vi "PeelingMXIDaily.vi"() -> ()   [LabVIEW 2012]
uses:
  <vilib>/addons/database/Connection.llb/DB Tools Open Connec (Path).vi
  <vilib>/addons/database/Connection.llb/Conn Execute.vi
  <vilib>/addons/database/Recordset.llb/Rec Fetch Recordset Data (R).vi
  <vilib>/addons/database/Recordset.llb/Rec Destroy - Connection.vi
  <vilib>/Utility/file.llb/Write To Spreadsheet File (string).vi
  <vilib>/addons/database/_DB Variant To Data/Database Variant To Data.xnode
  <vilib>/addons/database/NI_Database_API.lvlib
panel:
  out "error out":errorcluster
  out "Array 2":string[][](array[string])
  out "spreadsheet string":string
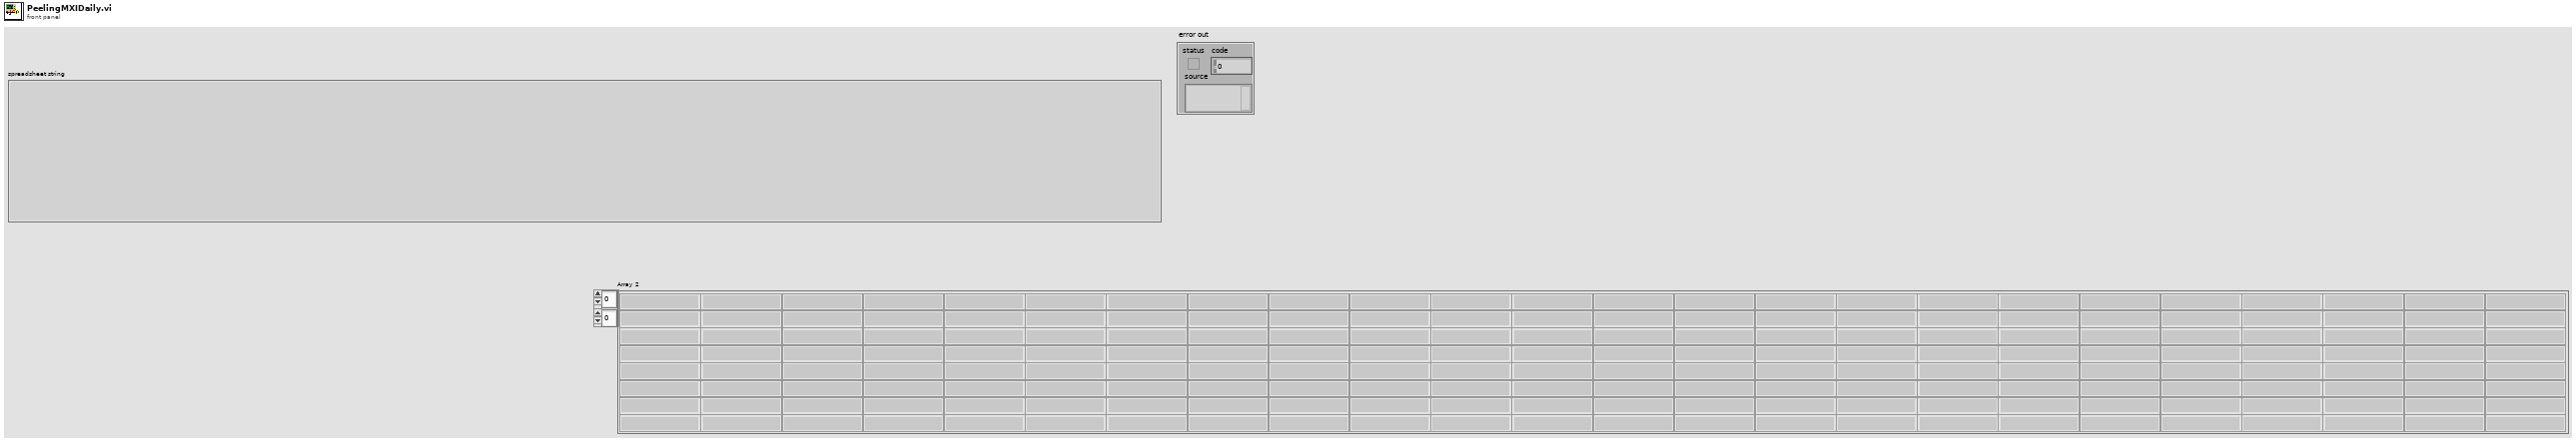
[diagram p1: front panel]
types:
  T1 = typedef "NI_Database_API.lvlib/Conn ObjectReference.ctl" = refnum<k1>
  T2 = typedef "NI_Database_API.lvlib/Rec ObjectReference.ctl" = refnum<k1>
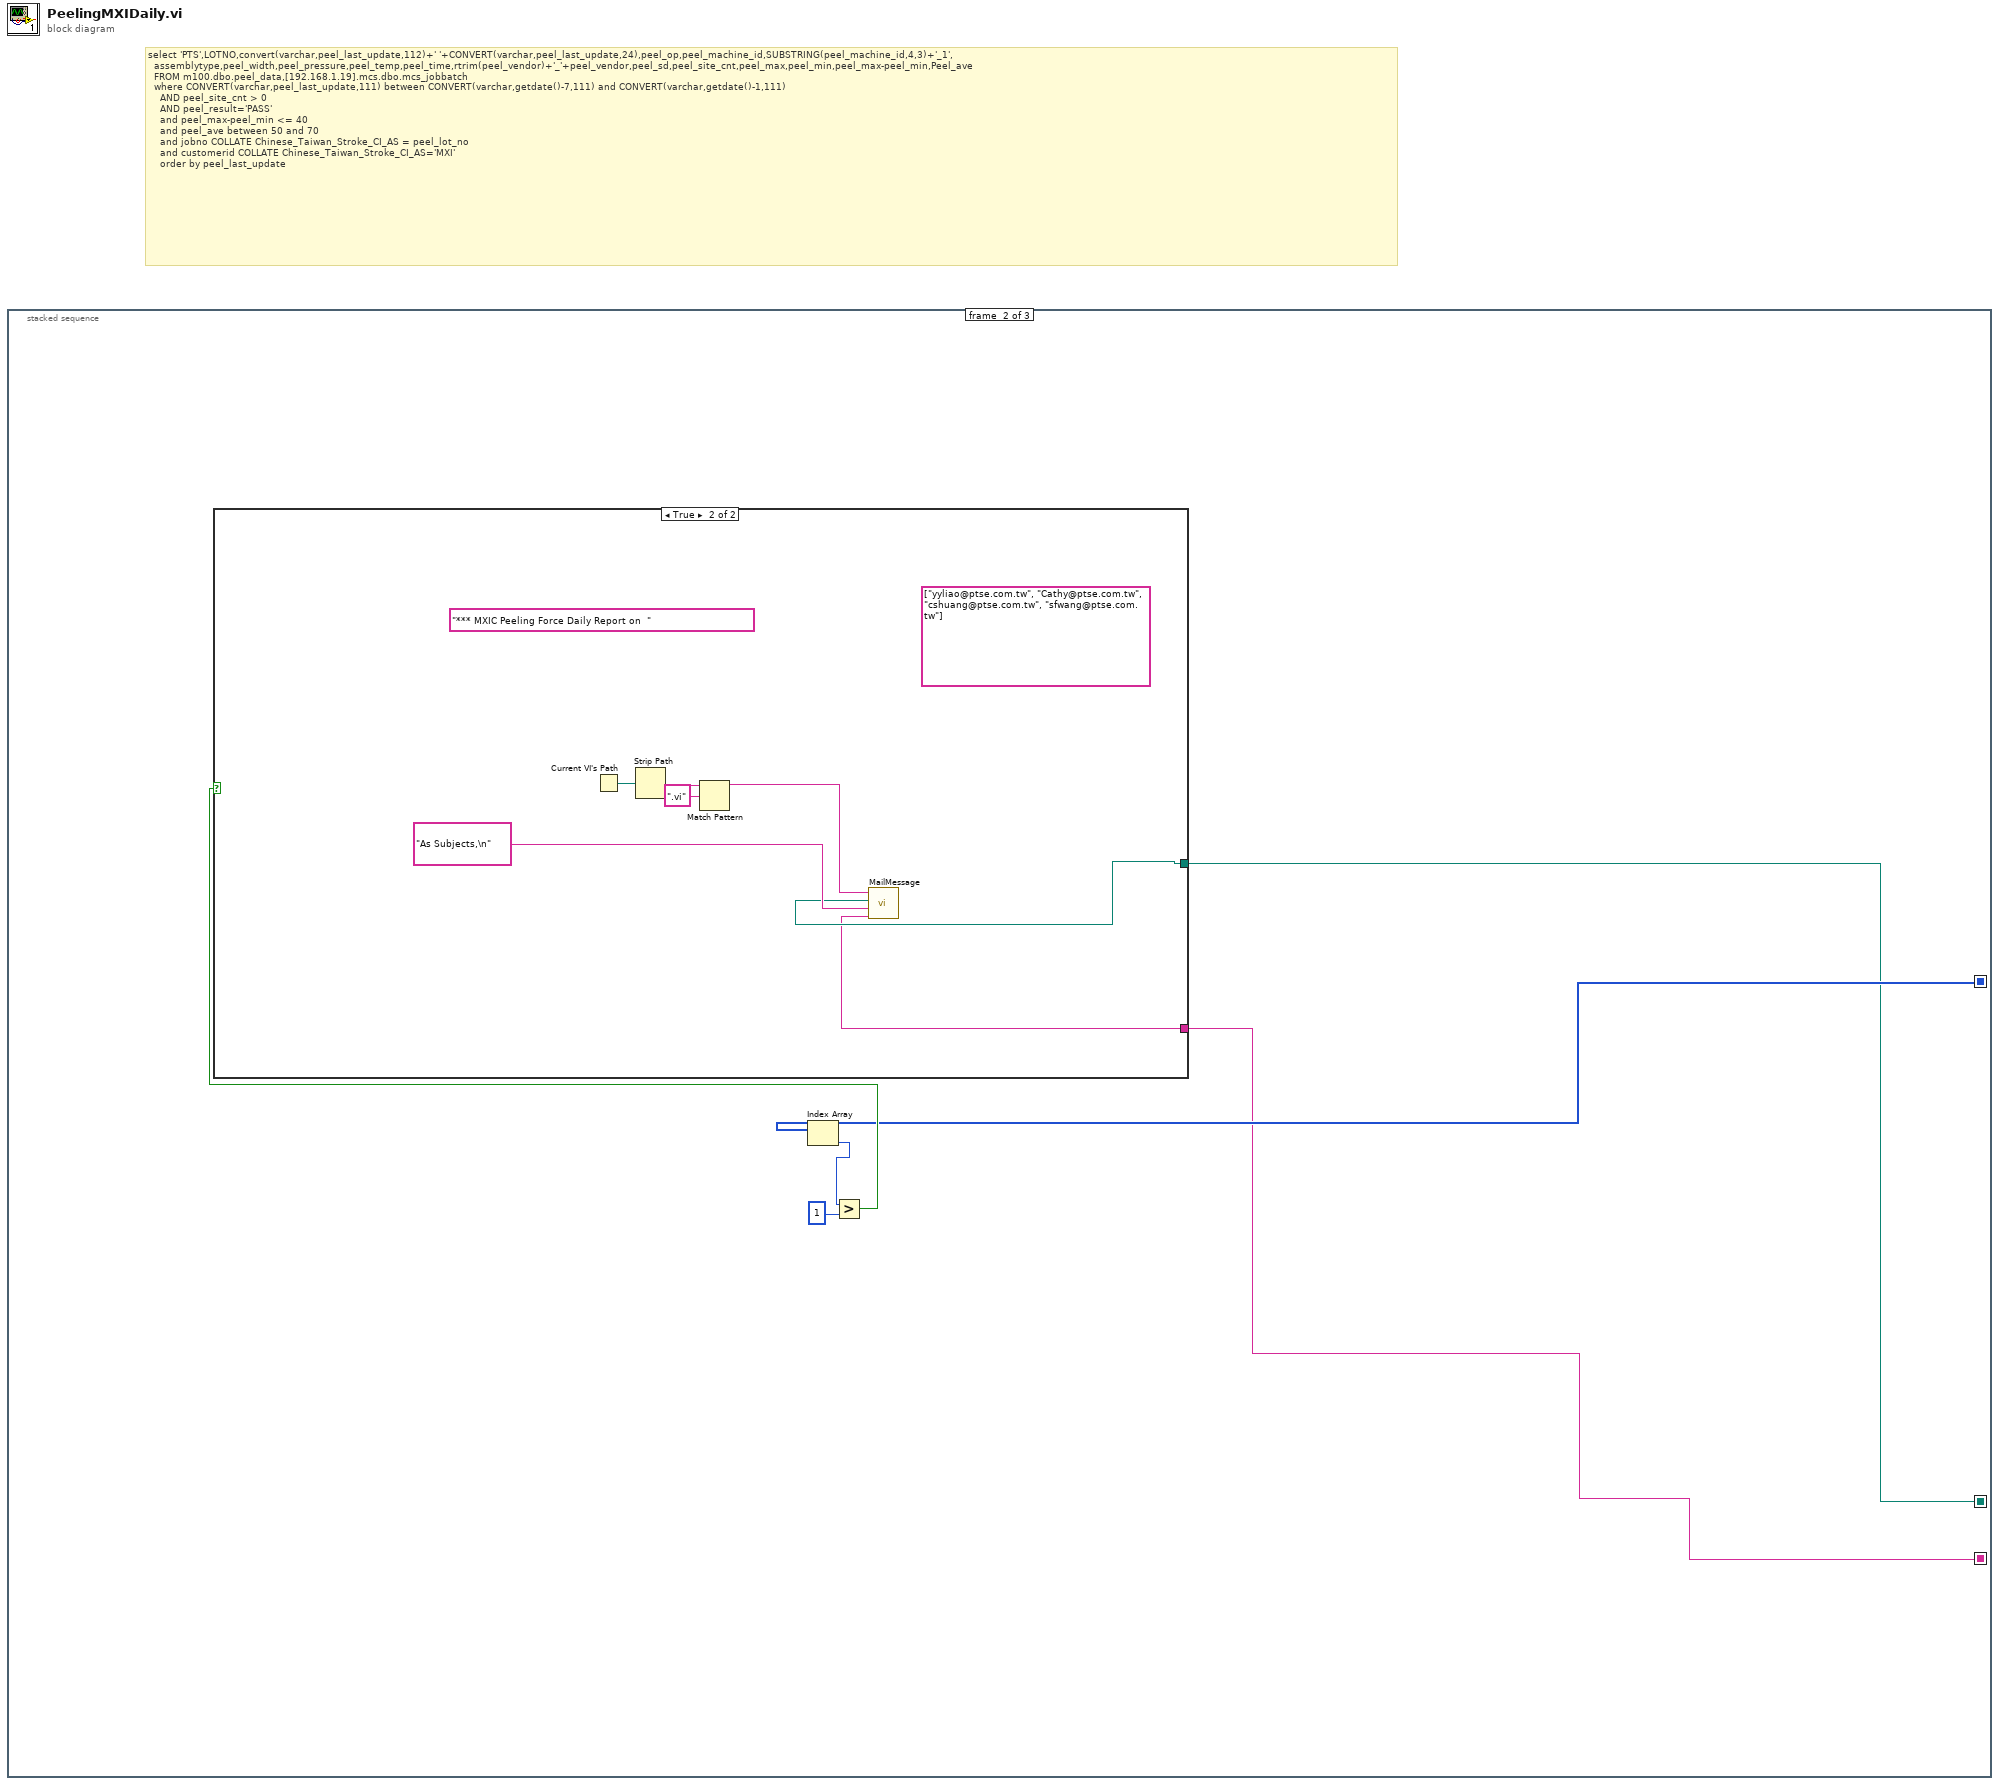
[diagram p0: block diagram]
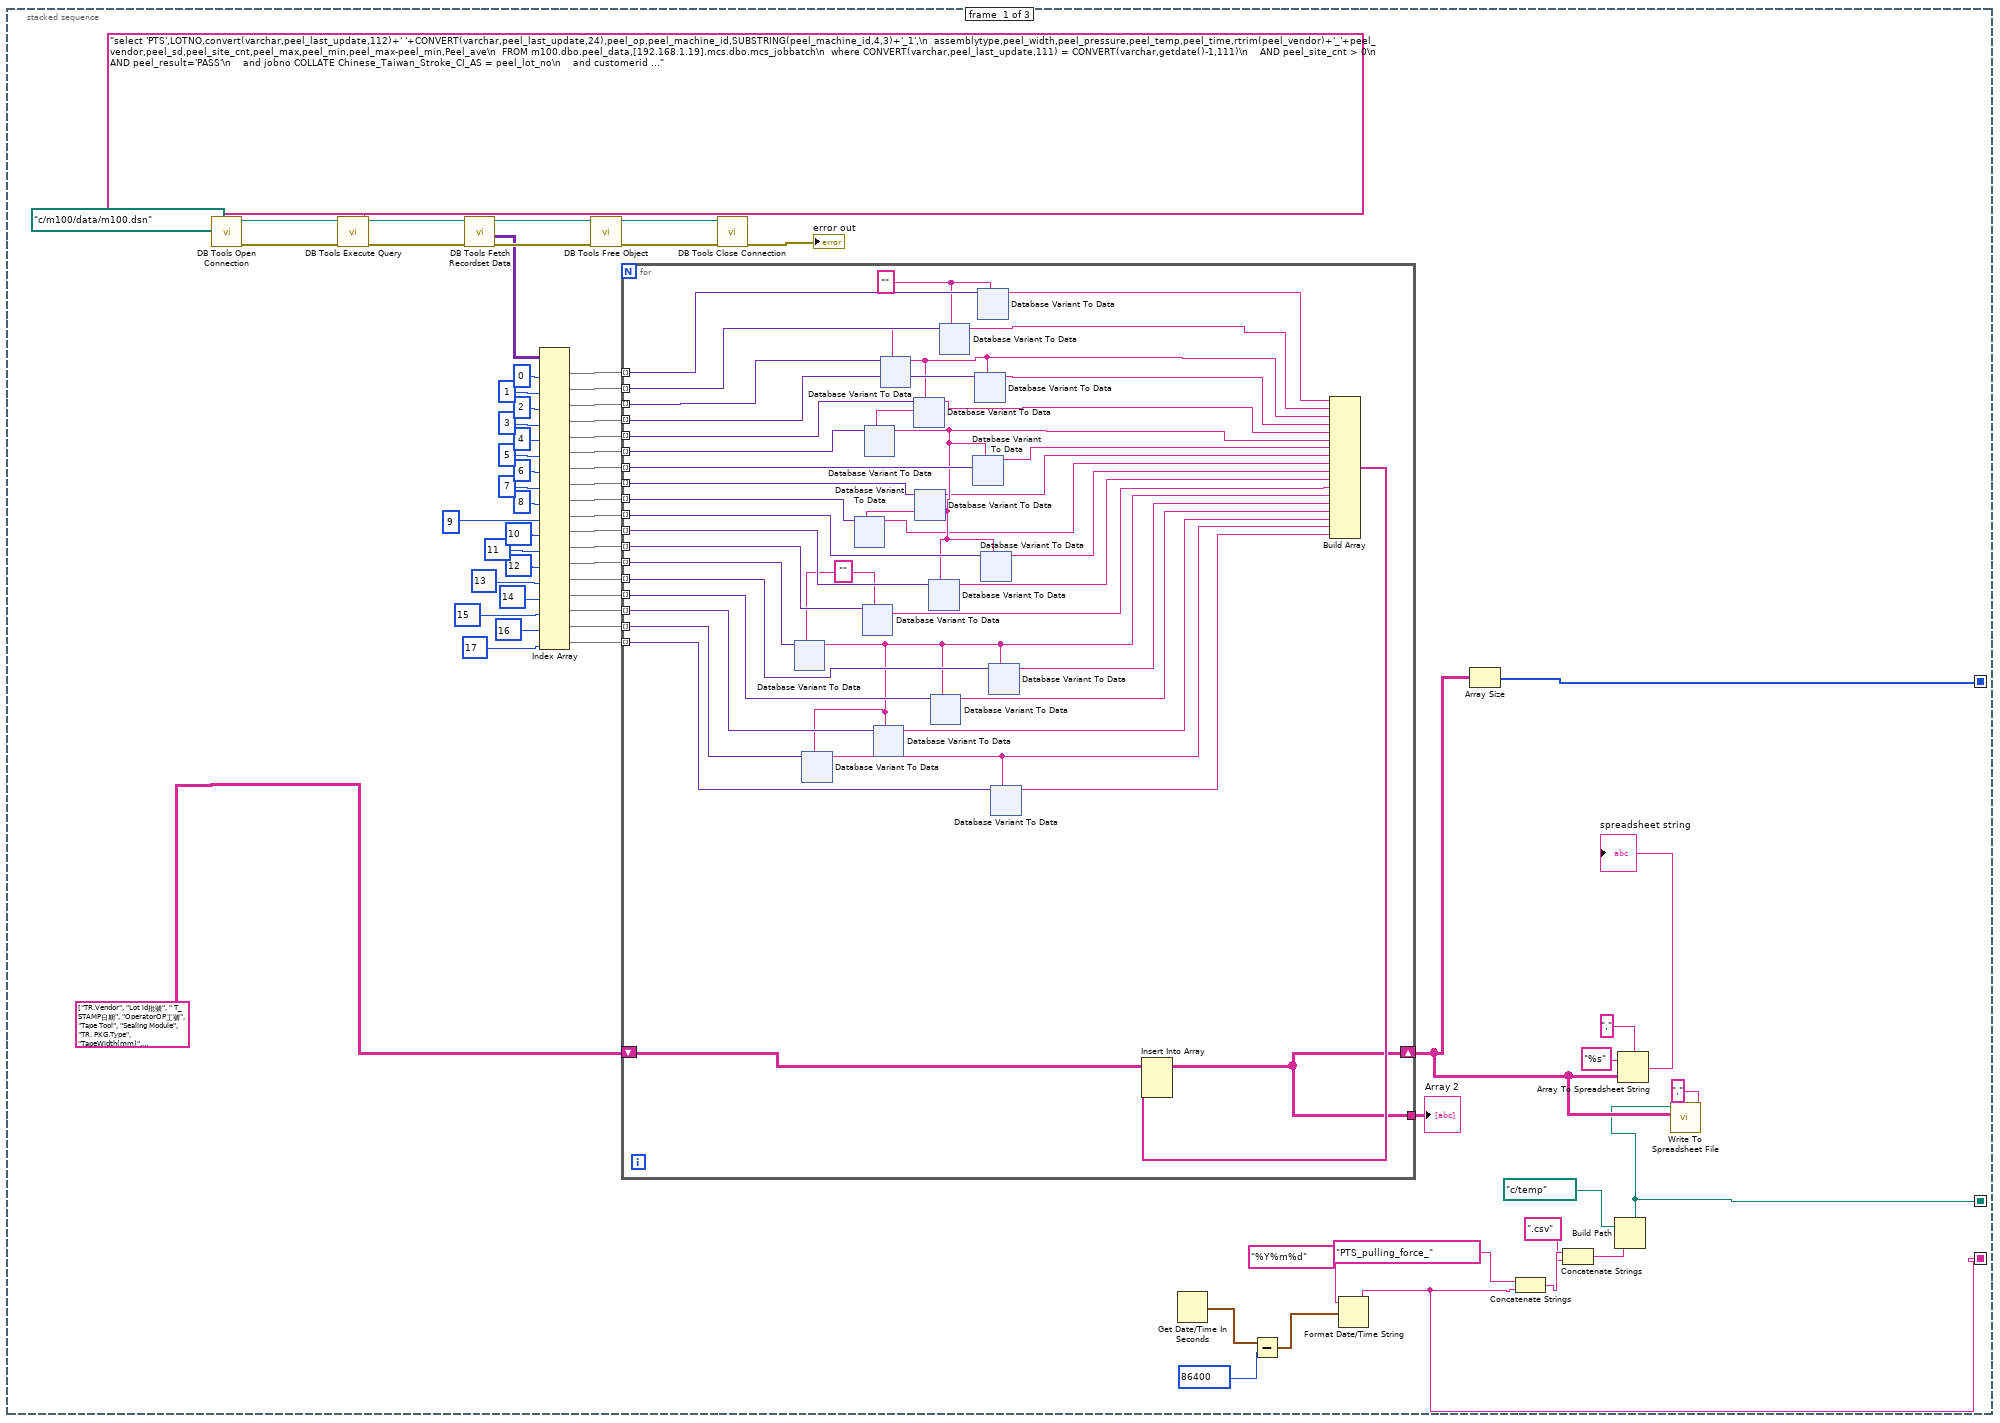
[diagram p2: hidden frame]
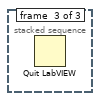
[diagram p4: hidden frame]
diagram:
  # "select 'PTS',LOTNO,convert(varchar,peel_last_update,112)+' '+CONVERT(varchar,peel_last_update,24),peel_op,peel_machine_id,SUBSTRING(peel_machine_id,4,3)+'_1',\n  assemblytype,peel_width,peel_pressure,peel_temp,peel_time,rtrim(peel_vendor)+'_'+peel_vendor,peel_sd,peel_site_cnt,peel_max,peel_min,peel_max-peel_min,Peel_ave\n  FROM m100.dbo.peel_data,[192.168.1.19].mcs.dbo.mcs_jobbatch\n  where CONVERT(varchar,peel_last_update,111) between CONVERT(varchar,getdate()-7,111) and CONVERT(varchar,getdate()-1,111)\n    AND peel_site_cnt > 0\n    AND peel_result='PASS'\n    and peel_max-peel_min <= 40\n    and peel_ave between 50 and 70\n    and jobno COLLATE Chinese_Taiwan_Stroke_CI_AS = peel_lot_no\n    and customerid COLLATE Chinese_Taiwan_Stroke_CI_AS='MXI'\n    order by peel_last_update"
  n1 = stacked-sequence {
    seq-local: [w35 _ _] -> [_ w687 _]
    seq-local: [w6 _ _] -> [_ w686 _]
    seq-local: [w2 _ _] -> [_ w685 _]
    frame #0 {
      n2 = call-poly <vilib>:"DB Tools Open Connection.vi"("connection information"=path "c:/m100/data/m100.dsn") -> ("error out"=w62:errorcluster, "connection reference"=w66:T1)  [unwired: 7 in]
      n3 = call-poly <vilib>:"DB Tools Execute Query.vi"("error in (no error)"=w62, "SQL query"="select 'PTS',LOTNO,convert(varchar,peel_last_update,112)+' '+CONVERT(varchar,peel_last_update,24),peel_op,peel_machine_id,SUBSTRING(peel_machine_id,4,3)+'_1',\n  assemblytype,peel_width,peel_pressure,peel_temp,peel_time,rtrim(peel_vendor)+'_'+peel_vendor,peel_sd,peel_site_cnt,peel_max,peel_min,peel_max-peel_min,Peel_ave\n  FROM m100.dbo.peel_data,[192.168.1.19].mcs.dbo.mcs_jobbatch\n  where CONVERT(varchar,peel_last_update,111) = CONVERT(varchar,getdate()-1,111)\n    AND peel_site_cnt > 0\n    AND peel_result='PASS'\n    and jobno COLLATE Chinese_Taiwan_Stroke_CI_AS = peel_lot_no\n    and customerid COLLATE Chinese_Taiwan_Stroke_CI_AS='MXI'\n    order by peel_last_update", "connection reference"=w66) -> ("error out"=w61:errorcluster, "recordset reference"=w65:T2)  [unwired: 5 in]
      n4 = call-poly <vilib>:"DB Tools Fetch Recordset Data.vi"("error in (no error)"=w61, "recordset reference"=w65) -> ("error out"=w60:errorcluster, "recordset data"=w29:variant[][], "recordset reference out"=w64:T2)  [unwired: 3 in]
      n5 = Index Array(array=w29, index (col) #1=0 ("disabled index (col)"), index (col) #2=1 ("index (col)"), index (col) #3=2 ("index (col)"), index (col) #4=3 ("index (col)"), index (col) #5=4 ("index (col)"), index (col) #6=5 ("index (col)"), index (col) #7=6 ("index (col)"), index (col) #8=7 ("index (col)"), index (col) #9=8 ("index (col)"), index (col) #10=9 ("index (col)"), index (col) #11=10 ("index (col)"), index (col) #12=11 ("index (col)"), index (col) #13=12 ("index (col)"), index (col) #14=13 ("index (col)"), index (col) #15=14 ("index (col)"), index (col) #16=15 ("index (col)"), index (col) #17=16 ("index (col)"), index (col) #18=17 ("index (col)")) -> (element #1=w46:variant[], element #2=w45:variant[], element #3=w44:variant[], element #4=w43:variant[], element #5=w42:variant[], element #6=w41:variant[], element #7=w40:variant[], element #8=w39:variant[], element #9=w38:variant[], element #10=w37:variant[], element #11=w36:variant[], element #12=w32:variant[], element #13=w31:variant[], element #14=w23:variant[], element #15=w22:variant[], element #16=w21:variant[], element #17=w20:variant[], element #18=w19:variant[])  [unwired: 18 in]
      n6 = call-poly <vilib>:"DB Tools Free Object.vi"("error in (no error)"=w60, "recordset reference"=w64) -> ("error out"=w59:errorcluster, "connection reference"=w63:T1)  [unwired: 8 in]
      n7 = for {
        tunnel: w46 -> [w108] mode=indexing
        tunnel: w45 -> [w107] mode=indexing
        tunnel: w44 -> [w106] mode=indexing
        tunnel: w43 -> [w105] mode=indexing
        tunnel: w42 -> [w104] mode=indexing
        tunnel: w41 -> [w103] mode=indexing
        tunnel: w40 -> [w102] mode=indexing
        tunnel: w39 -> [w101] mode=indexing
        tunnel: w38 -> [w100] mode=indexing
        tunnel: w37 -> [w99] mode=indexing
        tunnel: w36 -> [w98] mode=indexing
        tunnel: [w95] -> w18
        shift-right: [w95] -> w14
        shift-left: string[][] [["TR.Vendor", "Lot id批號", " T_STAMP日期", "OperatorOP工號", "Tape Tool", "Sealing Module", "TR. PKG.Type", "TapeWidth(mm)", "Pressure壓力(psi)", "Temp.溫度", "Dwell Time", "Cover.Carrier.Tape", "Average.Std(標準差)", "SiteCount(點數)", "Max最大值", "Min最小值", "Range最大-最小", "Average平均值"]] ("Array") -> [w94]
        tunnel: w32 -> [w93] mode=indexing
        tunnel: w31 -> [w92] mode=indexing
        tunnel: w23 -> [w78] mode=indexing
        tunnel: w22 -> [w77] mode=indexing
        tunnel: w21 -> [w76] mode=indexing
        tunnel: w20 -> [w75] mode=indexing
        tunnel: w19 -> [w74] mode=indexing
        w91 = ""
        w88 = ""
        n8 = xnode "Database Variant To Data"("database variant"=w92, "type"=w91) -> ("data"=w73:string)  [unwired: 1 in, 1 out]
        n9 = xnode "Database Variant To Data"("database variant"=w75, "type"=w73) -> ("data"=w68:string)  [unwired: 1 in, 1 out]
        n10 = xnode "Database Variant To Data"("database variant"=w93, "type"=w91) -> ("data"=w90:string)  [unwired: 1 in, 1 out]
        n11 = xnode "Database Variant To Data"("database variant"=w76, "type"=w73) -> ("data"=w70:string)  [unwired: 1 in, 1 out]
        n12 = xnode "Database Variant To Data"("database variant"=w106, "type"=w88) -> ("data"=w85:string)  [unwired: 1 in, 1 out]
        n13 = xnode "Database Variant To Data"("database variant"=w103, "type"=w85) -> ("data"=w84:string)  [unwired: 1 in, 1 out]
        n14 = xnode "Database Variant To Data"("database variant"=w100, "type"=w84) -> ("data"=w81:string)  [unwired: 1 in, 1 out]
        n15 = xnode "Database Variant To Data"("database variant"=w104, "type"=w85) -> ("data"=w86:string)  [unwired: 1 in, 1 out]
        n16 = xnode "Database Variant To Data"("database variant"=w101, "type"=w84) -> ("data"=w82:string)  [unwired: 1 in, 1 out]
        n17 = xnode "Database Variant To Data"("database variant"=w98, "type"=w84) -> ("data"=w79:string)  [unwired: 1 in, 1 out]
        n18 = xnode "Database Variant To Data"("database variant"=w77, "type"=w73) -> ("data"=w71:string)  [unwired: 1 in, 1 out]
        n19 = xnode "Database Variant To Data"("database variant"=w107, "type"=w88) -> ("data"=w89:string)  [unwired: 1 in, 1 out]
        n20 = xnode "Database Variant To Data"("database variant"=w102, "type"=w84) -> ("data"=w83:string)  [unwired: 1 in, 1 out]
        n21 = xnode "Database Variant To Data"("database variant"=w105, "type"=w85) -> ("data"=w87:string)  [unwired: 1 in, 1 out]
        n22 = xnode "Database Variant To Data"("database variant"=w108, "type"=w88) -> ("data"=w97:string)  [unwired: 1 in, 1 out]
        n23 = xnode "Database Variant To Data"("database variant"=w99, "type"=w84) -> ("data"=w80:string)  [unwired: 1 in, 1 out]
        n24 = xnode "Database Variant To Data"("database variant"=w78, "type"=w73) -> ("data"=w72:string)  [unwired: 1 in, 1 out]
        n25 = xnode "Database Variant To Data"("database variant"=w74, "type"=w68) -> ("data"=w69:string)  [unwired: 1 in, 1 out]
        n26 = Build Array(w97, w89, w85, w87, w86, w84, w83, w82, w81, w80, w79, w90, w73, w72, w71, w70, w68, w69) -> (w96:string[])
        n27 = Insert Into Array(array=w94, new element=w96) -> (w95:string[][])  [unwired: 2 in]
      }
      "Array 2" <- w18
      n28 = call <vilib>:"DB Tools Close Connection.vi"("error in (no error)"=w59, "connection reference"=w63) -> ("error out"=→"error out":errorcluster)  [unwired: 5 in]
      n29 = Get Date/Time In Seconds() -> (seconds since 1Jan1904=w5:timestamp)
      n30 = Subtract(x=w5, y=86400) -> (x-y=w3:timestamp)
      n31 = Format Date/Time String(time format string (%c)="%Y%m%d", seconds (now)=w3) -> (date/time string=w6:string)  [unwired: 1 in]
      n32 = Array Size(array=w14) -> (size(s)=w35:i32[])
      n33 = Concatenate Strings("PTS_pulling_force_" ("string"), w6) -> (w10:string)
      n34 = Concatenate Strings(w10, ".csv" ("string")) -> (w8:string)
      n35 = Build Path(base path=path "c:/temp", name or relative path=w8) -> (appended path=w2:path)
      n36 = Array To Spreadsheet String(delimiter (Tab)=",", array=w14, 3:"%s" ("format string")) -> (spreadsheet string=→"spreadsheet string":string)
      n37 = call-poly <vilib>:"Write To Spreadsheet File.vi"("delimiter (\\t)"="," ("delimiter (\\t)"), "2D data"=w14, "file path (dialog if empty)"=w2) -> ()  [unwired: 5 in, 1 out]
    }
    frame #1 {
      n38 = Index Array(array=w687) -> (element=w690:i32)  [unwired: 1 in]
      n39 = Greater?(x=w690, y=1) -> (0:w688:bool)
      n40 = case shown="True" w688 {
        tunnel: w685 -> [_ w692]
        tunnel: w686 -> [_ w691]
        frame False {
        }
        frame True {
          (unwired) string[] ["yyliao@ptse.com.tw", "Cathy@ptse.com.tw", "cshuang@ptse.com.tw", "sfwang@ptse.com.tw"] ("recipients")
          (unwired) "*** MXIC Peeling Force Daily Report on  " ("subject ([No Subject])")
          n41 = Current VI's Path() -> (path=w696:path)
          n42 = Strip Path(path=w696) -> (name=w695:string)  [unwired: 1 out]
          n43 = Match Pattern(string=w695, regular expression=".vi") -> (before substring=w693:string)  [unwired: 1 in, 3 out]
          n44 = call "MailMessage.vi"("AddSubject"=w691, "message"="As Subjects,\n", "file path"=w692, "program"=w693) -> ()  [unwired: 8 in]
        }
      }
    }
    frame #2 {
      n45 = Quit LabVIEW() -> ()  [unwired: 1 in]
    }
  }
